vi "ControlsToCommands.vi"(11 "input cluster":T1) -> (3 "output cluster":T2)   [LabVIEW 2016]
uses:
  ControlsToCommands.ctl
  Controls.ctl
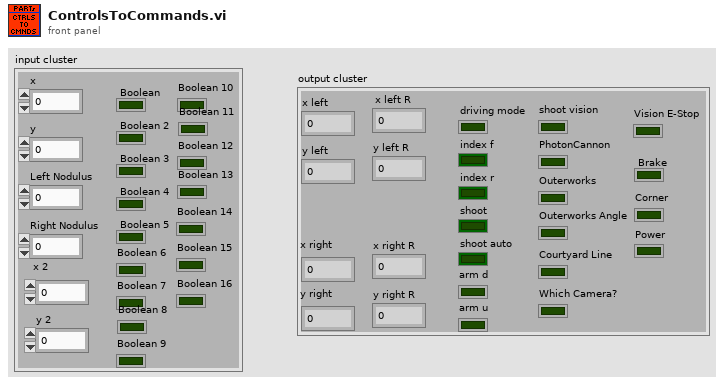
[diagram p1: front panel]
types:
  T1 = typedef "Controls.ctl" = cluster{"x":dbl, "y":dbl, "Left Nodulus":dbl, "Right Nodulus":dbl, "Boolean":bool, "Boolean 2":bool, "Boolean 3":bool, "Boolean 4":bool, "Boolean 5":bool, "Boolean 6":bool, "Boolean 7":bool, "Boolean 8":bool, "Boolean 9":bool, "Boolean 10":bool, "Boolean 11":bool, "Boolean 12":bool, "Boolean 13":bool, "Boolean 14":bool, "Boolean 15":bool, "x 2":dbl, "y 2":dbl, "Boolean 16":bool}
  T2 = typedef "ControlsToCommands.ctl" = cluster{"x left":dbl, "y left":dbl, "x right":dbl, "y right":dbl, "driving mode":bool, "index f":bool, "index r":bool, "shoot":bool, "shoot auto":bool, "arm d":bool, "arm u":bool, "shoot vision":bool, "PhotonCannon":bool, "Outerworks":bool, "Outerworks Angle":bool, "Courtyard Line":bool, "Which Camera?":bool, "Vision E-Stop":bool, "x left R":dbl, "y left R":dbl, "x right R":dbl, "y right R":dbl, "Brake":bool, "Corner":bool, "Power":bool}
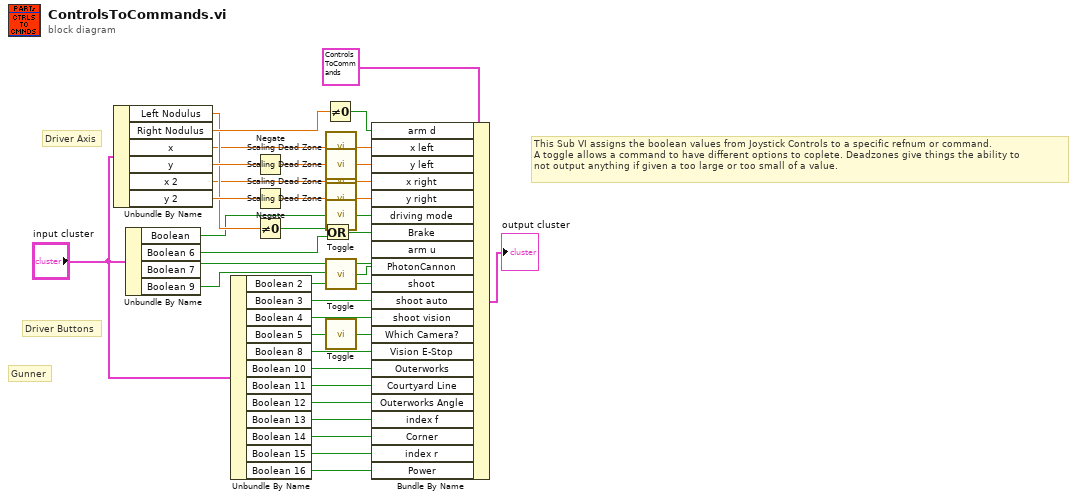
[diagram p0: block diagram]
diagram:
  # "This Sub VI assigns the boolean values from Joystick Controls to a specific refnum or command.\nA toggle allows a command to have different options to coplete. Deadzones give things the ability to \nnot output anything if given a too large or too small of a value."
  # "Driver Buttons"
  # "Gunner"
  # "Driver Axis"
  n1 = Unbundle By Name("input cluster") -> ("Left Nodulus"=w27:dbl, "Right Nodulus"=w29:dbl, "x"=w8:dbl, "y"=w36:dbl, "x 2"=w3:dbl, "y 2"=w35:dbl)
  n2 = Unbundle By Name("input cluster") -> ("Boolean"=w10:bool, "Boolean 6"=w25:bool, "Boolean 7"=w34:bool, "Boolean 9"=w33:bool)
  n3 = Unbundle By Name("input cluster") -> ("Boolean 2"=w23:bool, "Boolean 3"=w22:bool, "Boolean 4"=w21:bool, "Boolean 5"=w12:bool, "Boolean 8"=w20:bool, "Boolean 10"=w19:bool, "Boolean 11"=w18:bool, "Boolean 12"=w17:bool, "Boolean 13"=w16:bool, "Boolean 14"=w15:bool, "Boolean 15"=w14:bool, "Boolean 16"=w1:bool)
  n4 = Negate(x=w36) -> (-x=w9:dbl)
  n5 = Negate(x=w35) -> (-x=w6:dbl)
  n6 = Not Equal To 0?(x=w27) -> (x != 0?=w26:bool)
  n7 = Or(x=w26, y=w25) -> (x .or. y?=w24:bool)
  n8 = Not Equal To 0?(x=w29) -> (x != 0?=w28:bool)
  n9 = call "Scaling Dead Zone.vi"("Input"=w8) -> ("Output"=w7:dbl)  [unwired: 4 in]
  n10 = call "Scaling Dead Zone.vi"("Input"=w9) -> ("Output"=w4:dbl)  [unwired: 4 in]
  n11 = call "Scaling Dead Zone.vi"("Input"=w3) -> ("Output"=w2:dbl)  [unwired: 4 in]
  n12 = call "Scaling Dead Zone.vi"("Input"=w6) -> ("Output"=w5:dbl)  [unwired: 4 in]
  n13 = call "Toggle.vi"("Input"=w10) -> ("Output"=w11:bool)  [unwired: 4 in]
  n14 = call "Toggle.vi"("Input"=w33) -> ("Output"=w32:bool)  [unwired: 4 in]
  n15 = call "Toggle.vi"("Input"=w12) -> ("Output"=w13:bool)  [unwired: 4 in]
  n16 = Bundle By Name(cluster=T2 {"x left"=0.0, "y left"=0.0, "x right"=0.0, "y right"=0.0, "driving mode"=FALSE, "index f"=FALSE, "index r"=FALSE, "shoot"=FALSE, "shoot auto"=FALSE, "arm d"=FALSE, "arm u"=FALSE, "shoot vision"=FALSE, "PhotonCannon"=FALSE, "Outerworks"=FALSE, "Outerworks Angle"=FALSE, "Courtyard Line"=FALSE, "Which Camera?"=FALSE, "Vision E-Stop"=FALSE, "x left R"=0.0, "y left R"=0.0, "x right R"=0.0, "y right R"=0.0, "Brake"=FALSE, "Corner"=FALSE, "Power"=FALSE} ("input cluster"), "arm d"=w28, "x left"=w7, "y left"=w4, "x right"=w2, "y right"=w5, "driving mode"=w11, "Brake"=w24, "arm u"=w34, "PhotonCannon"=w32, "shoot"=w23, "shoot auto"=w22, "shoot vision"=w21, "Which Camera?"=w13, "Vision E-Stop"=w20, "Outerworks"=w19, "Courtyard Line"=w18, "Outerworks Angle"=w17, "index f"=w16, "Corner"=w15, "index r"=w14, "Power"=w1) -> (→"output cluster":T2)
